vi "Set Channel (Blue).vi"(8 "error in (no error)":errorcluster, 10 "Channel Data":T1, 11 "ARGB Image":T2) -> (0 "error out":errorcluster, 3 "ARGB Image (Duplicate)":T2)   [LabVIEW 2020, in "g_ar_toolkit.image.lvlib"]
uses:
  g_ar_toolkit.image.lvlib
  ARGB Image.ctl
  Greyscale Image.ctl
  ARGBChannels.ctl
  g_ar_toolkit.common/Module Path.vi
  <vilib>/Utility/error.llb/Error Cluster From Error Code.vi
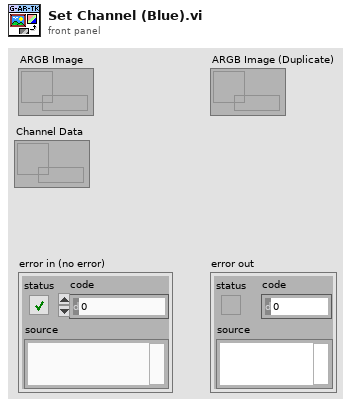
[diagram p1: front panel]
types:
  T1 = typedef "g_ar_toolkit.image.lvlib/Greyscale Image.ctl" = refnum<data-value>
  T2 = typedef "g_ar_toolkit.image.lvlib/ARGB Image.ctl" = refnum<data-value>
  T3 = typedef "g_ar_toolkit.image.lvlib/ARGBChannels.ctl" = enum8{"Blue", "Green", "Red", "Alpha"}
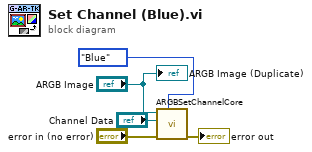
[diagram p0: block diagram]
diagram:
  n1 = call "ARGBSetChannelCore.vi"("Channels"=ARGBChannels."Blue" ("Extract_Operation"), "error in (no error)"="error in (no error)", "Channel Data"="Channel Data", "Image"="ARGB Image") -> ("error out"=→"error out":errorcluster)  [unwired: 7 in]
  "ARGB Image (Duplicate)" <- "ARGB Image"
